vi "Test Manager Initialized.vi"(8 "error in (no error)":errorcluster, 11 "Test Manager Interface in":refnum<class "Test Manager Interface.lvclass">) -> (0 "error out":errorcluster, 3 "Test Manager Interface out":refnum<class "Test Manager Interface.lvclass">)   [LabVIEW 2020, in "Test Manager Interface.lvlib" / "Test Manager Interface.lvclass"]
uses:
  Test Manager Interface.lvclass
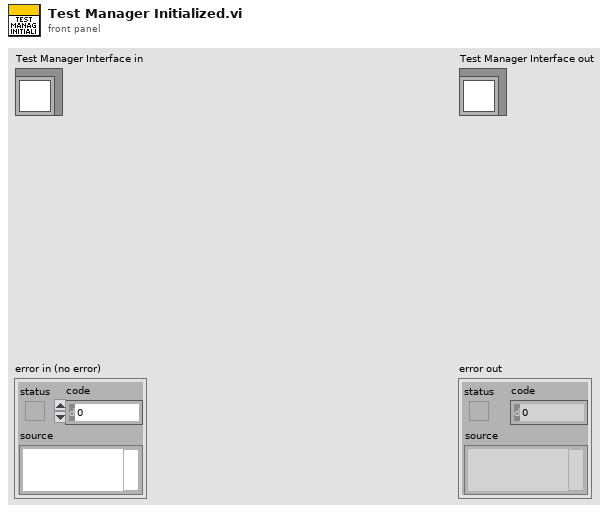
[diagram p1: front panel]
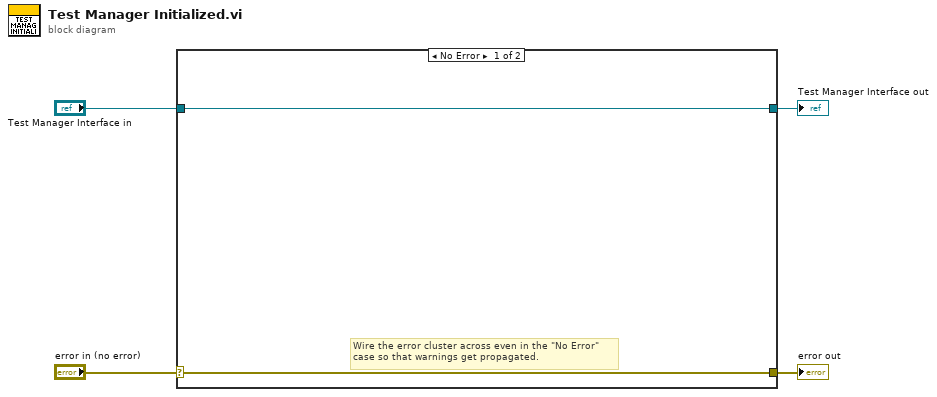
[diagram p0: block diagram]
diagram:
  n1 = case shown="No Error" "error in (no error)" {
    selector: "error in (no error)" -> [w5 w8]
    tunnel: [w5 w8] -> w3
    tunnel: [w6 w7] -> w1
    tunnel: "Test Manager Interface in" -> [w6 w7]
    frame No Error {
      # "Wire the error cluster across even in the \"No Error\"\ncase so that warnings get propagated."
    }
    frame Error {
    }
  }
  "error out" <- w3
  "Test Manager Interface out" <- w1
